vi "Pot To Arm Angle.vi"(1 "simulatedArmPot":dbl, 2 "potValueForArmAtZeroDegrees (pot value)":dbl) -> (0 "Numeric":sgl)   [LabVIEW 2017]
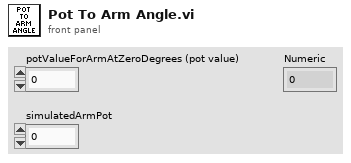
[diagram p1: front panel]
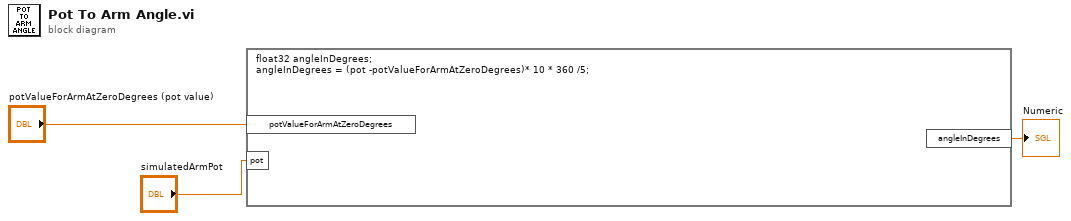
[diagram p0: block diagram]
diagram:
  n1 = formula code="float32 angleInDegrees;\nangleInDegrees = (pot -potValueForArmAtZeroDegrees)* 10 * 360 /5;"("pot"="simulatedArmPot", "potValueForArmAtZeroDegrees"="potValueForArmAtZeroDegrees (pot value)") -> ("angleInDegrees"=→"Numeric":sgl)
